vi "Untitled 1.vi"() -> ()   [LabVIEW 2018]
panel:
  out "Yaw":cluster{"X":dbl, "Y":dbl}[](graph)
  out "Pitch":cluster{"X":dbl, "Y":dbl}[](graph)
  out "Roll":cluster{"X":dbl, "Y":dbl}[](graph)
  in  "Simulation Time(sec)":dbl
  in  "Mass (Kg)":dbl
  in  "COG (m)":dbl[](array[numeric])
  in  "MOI (Kg/m^2)":dbl[][][](array[numeric])
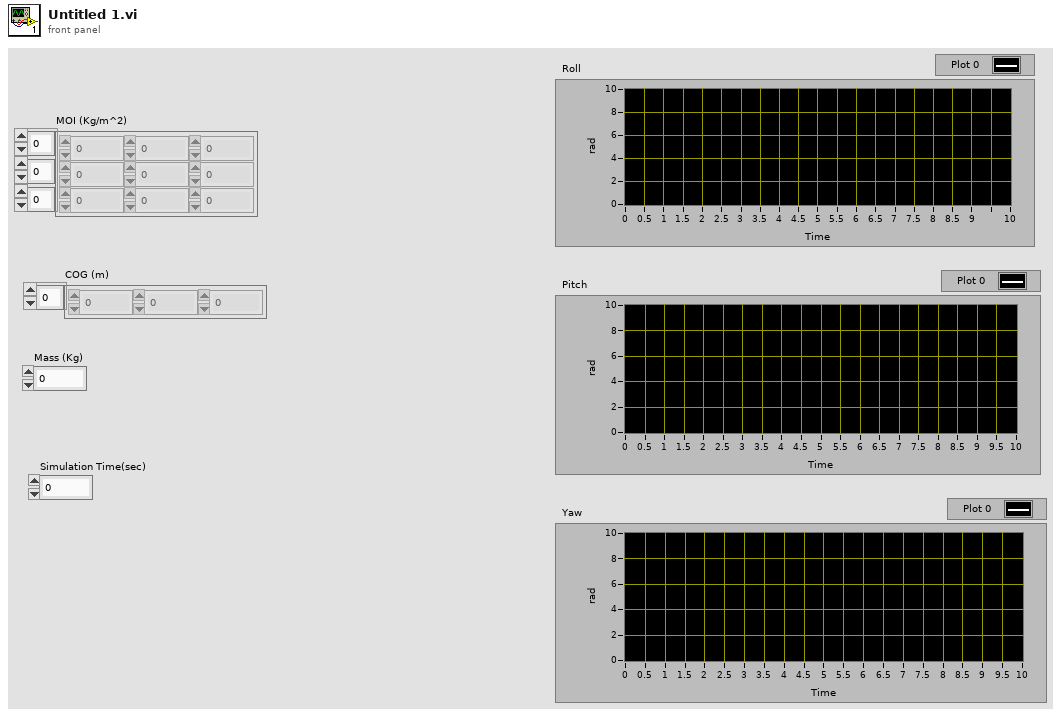
[diagram p1: front panel]
types:
  T1 = typedef "NI_Matrix.lvlib/RealMatrix.ctl" = dbl[][]
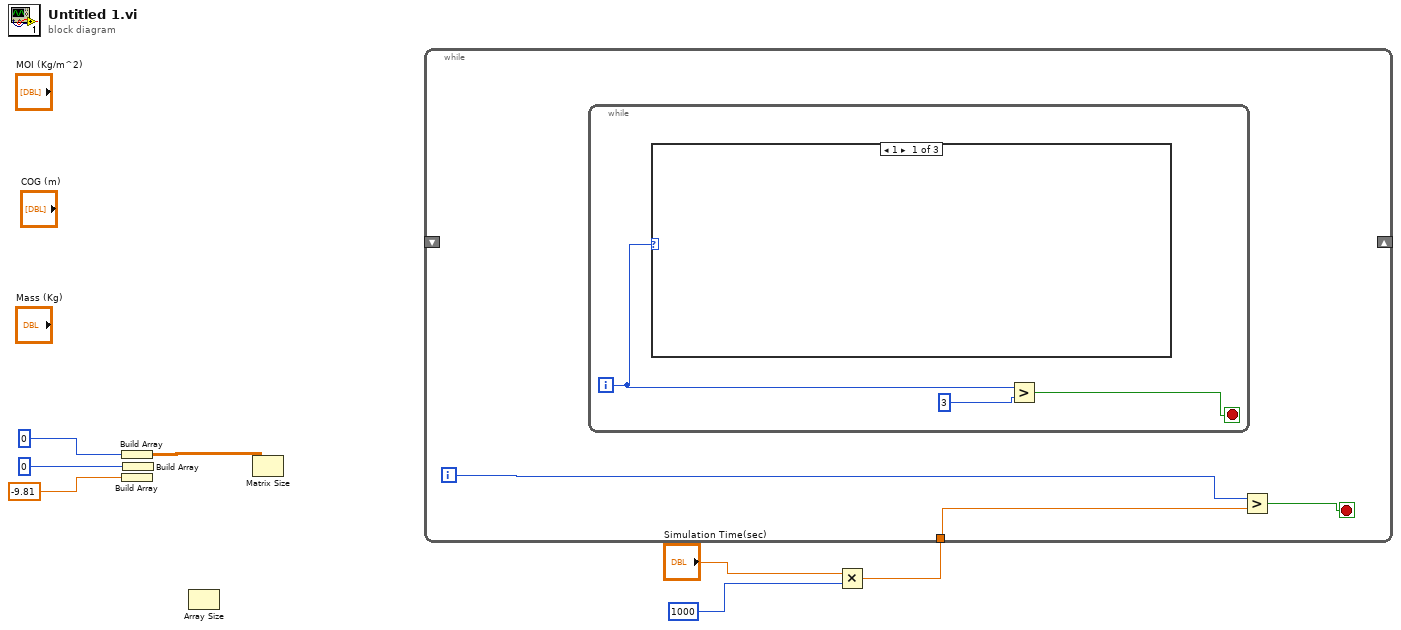
[diagram p0: block diagram]
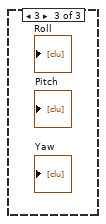
[diagram p3: hidden frame]
diagram:
  n1 = Build Array(0) -> (w1:T1)
  n2 = Build Array(-9.81) -> ()  [unwired: 1 out]
  n3 = Build Array(0) -> ()  [unwired: 1 out]
  n4 = Array Size() -> ()  [unwired: 1 in, 1 out]
  n5 = Matrix Size(0:w1) -> ()  [unwired: 2 out]
  n6 = Multiply(x="Simulation Time(sec)", y=1000) -> (x*y=w5:dbl)
  n7 = while {
    tunnel: w5 -> [w8]
    shift-right: _ -> [_]
    shift-left: _ -> [_]
    i -> [w9]
    stop <- w10 stop-if-true
    n8 = while {
      i -> [w11]
      stop <- w13 stop-if-true
      n9 = case shown="1" w11 {
        frame 1 {
        }
        frame 2 {
        }
        frame 3 {
        }
      }
      n10 = Greater?(x=w11, y=3) -> (0:w13:bool)
    }
    n11 = Greater?(x=w9, y=w8) -> (0:w10:bool)
  }
